vi "Wax Service.vi"(8 "error in (no error)":errorcluster, 11 "Manejo Turnos in":refnum<class "Manejo Turnos.lvclass">) -> (0 "error out":errorcluster, 3 "Manejo Turnos out":refnum<class "Manejo Turnos.lvclass">)   [LabVIEW 2020, in "Manejo Turnos.lvlib" / "Manejo Turnos.lvclass"]
uses:
  Manejo Turnos.lvclass
  C:/Program Files (x86)/National Instruments/LabVIEW 2020/vi.lib/ActorFramework/Actor/Actor.lvclass
  Manejo Turnos.lvclass/Manejo Turnos.ctl
  <vilib>/ActorFramework/Actor/Actor.lvclass/Actor.ctl
  User Interface Messages/Service to micros Msg/Service to micros Msg.lvclass/Service to micros Msg.ctl
  <vilib>/ActorFramework/Message Enqueuer/Message Enqueuer.lvclass/Message Enqueuer.ctl
  Manejo Turnos Messages/Delete Service Msg/Delete Service Msg.lvclass/Delete Service Msg.ctl
  <vilib>/ActorFramework/Message Enqueuer/Enqueue.vi
  <vilib>/ActorFramework/Message Enqueuer/Init from Existing Queue.vi
  User Interface Messages/Service to micros Msg/Service to micros Msg.lvclass
  C:/Program Files (x86)/National Instruments/LabVIEW 2020/vi.lib/ActorFramework/Message/Message.lvclass
  Manejo Turnos Messages/Delete Service Msg/Delete Service Msg.lvclass
  <vilib>/ActorFramework/Message Priority Queue/Priority Enqueue.vi
  <vilib>/ActorFramework/Message Enqueuer/Message Enqueuer.lvclass
  <vilib>/ActorFramework/Actor/Actor.lvclass
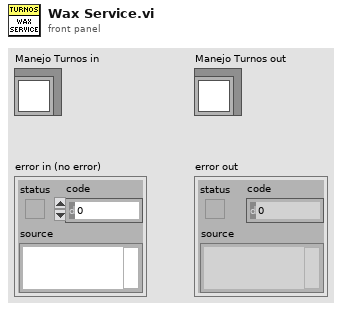
[diagram p1: front panel]
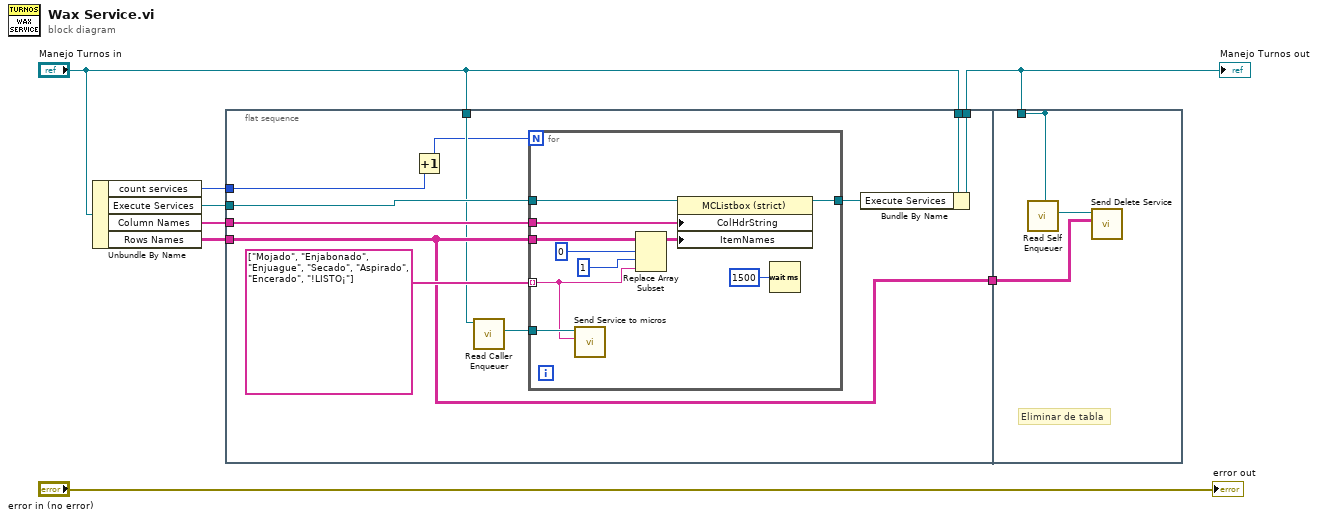
[diagram p0: block diagram]
diagram:
  n1 = Unbundle By Name("Manejo Turnos in") -> ("count services"=w2:i32, "Execute Services"=w6:refnum<vi>, "Column Names"=w5:string[], "Rows Names"=w4:string[][])
  n2 = flat-sequence {
    tunnel: w6 -> [w18]
    tunnel: w5 -> [w17]
    tunnel: [w15] -> w3
    tunnel: "Manejo Turnos in" -> [w14]
    tunnel: w4 -> [w13]
    tunnel: [w13] -> w7
    tunnel: w2 -> [w12]
    tunnel: "Manejo Turnos in" -> [w11]
    tunnel: [w30] -> _
    tunnel: w7 -> [w31]
    tunnel: w3 -> [w30]
    frame #0 {
      n3 = Increment(x=w12) -> (x+1=w9:i32)
      n4 = call <vilib>:"Read Caller Enqueuer.vi"("Actor"=w11) -> ("Caller Enqueuer"=w10:refnum<class "Message Enqueuer.lvclass">)  [unwired: 10 in]
      n5 = for {
        N: w9 -> [_]
        tunnel: string[] ["Mojado", "Enjabonado", "Enjuague", "Secado", "Aspirado", "Encerado", "!LISTO¡"] -> [w20] mode=indexing
        tunnel: w13 -> [w29]
        tunnel: w18 -> [w25]
        tunnel: w17 -> [w24]
        tunnel: [w23] -> w16
        tunnel: w10 -> [w21]
        n6 = call "Send Service to micros.vi"("Caracter"=w20, "Message Enqueuer"=w21) -> ()  [unwired: 8 in, 2 out]
        n7 = Replace Array Subset(array=w29, new element=w20, index (row)=0 ("index"), index (col)=1 ("disabled index (col)")) -> (w22:string[][])
        n8 = property class="MCListbox (strict)"(reference=w25, "ColHdrString"=w24, "ItemNames"=w22) -> (reference out=w23:refnum<vi>)  [unwired: 1 in, 1 out]
        n9 = Wait (ms)(milliseconds to wait=u32 1500) -> ()  [unwired: 1 out]
      }
      n10 = Bundle By Name(cluster=w14, "Execute Services"=w16) -> (w15:refnum<class "Manejo Turnos.lvclass">)
    }
    frame #1 {
      # "Eliminar de tabla"
      n11 = call <vilib>:"Read Self Enqueuer.vi"("Actor"=w30) -> ("Self Enqueuer"=w32:refnum<class "Message Enqueuer.lvclass">)  [unwired: 10 in]
      n12 = call "Send Delete Service.vi"("Service Name"=w31, "Message Enqueuer"=w32) -> ()  [unwired: 8 in, 2 out]
    }
  }
  "error out" <- "error in (no error)"
  "Manejo Turnos out" <- w3
